vi "Color Picker_ENQUE Cmds.vi"(7 "Add To Begining":bool, 8 "Error":errorcluster, 10 "Array":T1[](array[typedef]), 11 "Queue":refnum<queue>) -> (0 "Error Out":errorcluster)   [LabVIEW 2009]
doc: "Enques commands for the color picker program"
uses:
  Color Picker Controls/Color Picker_Cluster Command Data Set.ctl
  Color Picker Controls/Color Picker_ENUM Commands.ctl
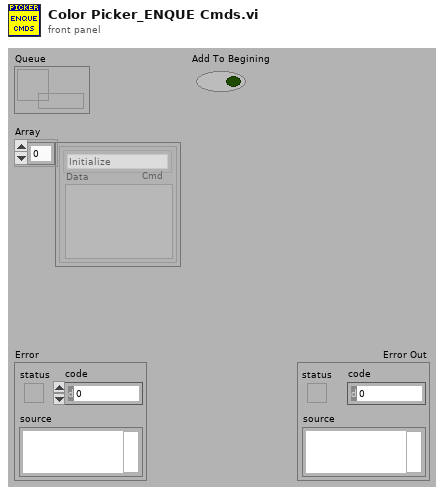
[diagram p1: front panel]
types:
  T1 = typedef "Color Picker_Cluster Command Data Set.ctl" = cluster{"Cmd":T2, "Data":variant}
  T2 = typedef "Color Picker_ENUM Commands.ctl" = enum16{"No Command", "Initialize", "Display Color", "Set Position", "Enable FP", "Hide FP", "Stop Program", "Set Original Color"}
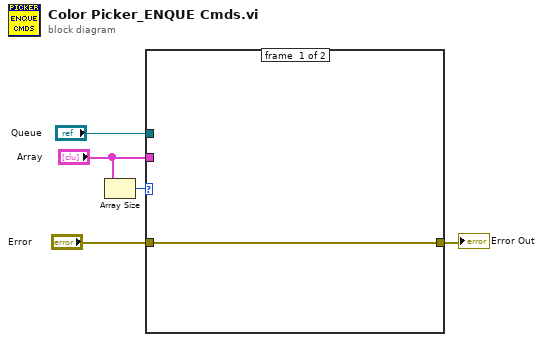
[diagram p0: block diagram]
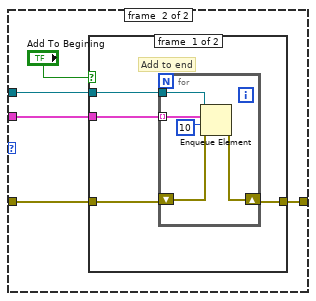
[diagram p2: hidden frame]
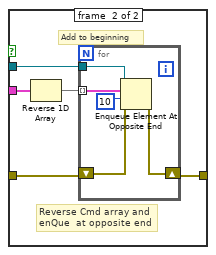
[diagram p3: hidden frame]
diagram:
  n1 = Array Size(array="Array") -> (size(s)=w5:i32)
  n2 = case shown="Default" w5 {
    tunnel: "Queue" -> [_ w11]
    tunnel: [w6 w10] -> w2
    tunnel: "Error" -> [w6 w9]
    tunnel: "Array" -> [_ w8]
    frame #0 {
    }
    frame #1 {
      n3 = case shown="True" "Add To Begining" {
        tunnel: w11 -> [w15 w25]
        tunnel: [w14 w24] -> w10
        tunnel: w9 -> [w13 w23]
        tunnel: w8 -> [w12 w22]
        frame #0 {
          # "Add to end"
          n4 = for {
            tunnel: w15 -> [w20]
            shift-right: [w18] -> w14
            shift-left: w13 -> [w19]
            tunnel: w12 -> [w17] mode=indexing
            n5 = Enqueue Element(queue=w20, element=w17, timeout in ms (-1)=10, error in (no error)=w19) -> (error out=w18:errorcluster)  [unwired: 2 out]
          }
        }
        frame #1 {
          # "Add to beginning"
          # "Reverse Cmd array and \nenQue  at opposite end"
          n6 = Reverse 1D Array(array=w22) -> (reversed array=w21:T1[])
          n7 = for {
            tunnel: w25 -> [w30]
            shift-right: [w28] -> w24
            shift-left: w23 -> [w29]
            tunnel: w21 -> [w27] mode=indexing
            n8 = Enqueue Element At Opposite End(queue=w30, element=w27, timeout in ms (-1)=10, error in (no error)=w29) -> (error out=w28:errorcluster)  [unwired: 2 out]
          }
        }
      }
    }
  }
  "Error Out" <- w2
